vi "dynamischeFarbe.vi"(9 "Boolesch":bool, 10 "Registerkarte":enum32{"Seite 2"}(tab)) -> ()   [LabVIEW 2017]
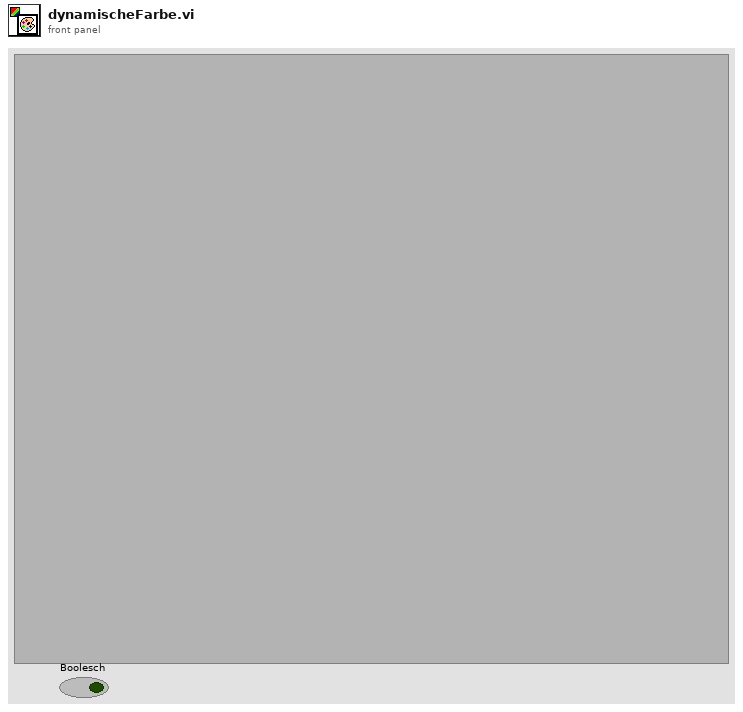
[diagram p1: front panel]
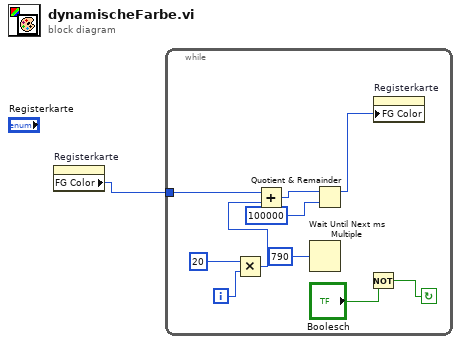
[diagram p0: block diagram]
diagram:
  n1 = property on="Registerkarte" class="RKElem (strikt)"() -> ("FG Color"=w1:u32)  [unwired: 2 in, 2 out]
  n2 = while {
    tunnel: w1 -> [w6]
    i -> [w8]
    stop <- w2 continue-if-true
    n3 = Multiply(x=20, y=w8) -> (x*y=w7:i32)
    n4 = Add(x=w6, y=w7) -> (x+y=w11:u32)
    n5 = Wait Until Next ms Multiple(millisecond multiple=u32 790 ("ms")) -> ()  [unwired: 1 out]
    n6 = Quotient & Remainder(x=w11, y=u32 100000) -> (x-y*floor(x/y)=w9:u32)  [unwired: 1 out]
    n7 = Not(x="Boolesch") -> (.not. x?=w2:bool)
    n8 = property on="Registerkarte" class="RKElem (strikt)"("FG Color"=w9) -> ()  [unwired: 2 in, 2 out]
  }
